vi "Final.vi"() -> ()   [LabVIEW 2013]
uses:
  <vilib>/DAQmx/read.llb/DAQmx Read (Analog Wfm 1Chan NSamp).vi
  <vilib>/DAQmx/miscellaneous.llb/DAQmx Fill In Error Info.vi
  <vilib>/express/express analysis/Spectral/Block/exnSpectralBlock spectral measurements PSD poly.vi
  <vilib>/express/express analysis/Spectral/Block/exnSpectralBlock spectral measurements PSD WFM.vi
  <vilib>/express/express analysis/Spectral/XNode/ExpressSpectralMeasurementsBlockNode.xnode
panel:
  in  "Signal de Reference":T1(ring)
  in  "Offset":dbl
  in  "Amplitude":dbl
  in  "Phase":dbl
  in  "Frequence 2":dbl
  in  "Voie physique DAQmx":tag="sHIT/ai0"
  in  "Statistiques":bool
  out "Moyenne":dbl
  out "Valeur eff":dbl
  out "Frequence":dbl
  in  "FFT":bool
  in  "Fenetre d'affichage (s)":dbl step=0.001
  out "Signal":waveform(dbl)[](graph)
  out "FFT":cluster{"f0":dbl, "df":dbl, "magnitude":dbl[]}(graph)
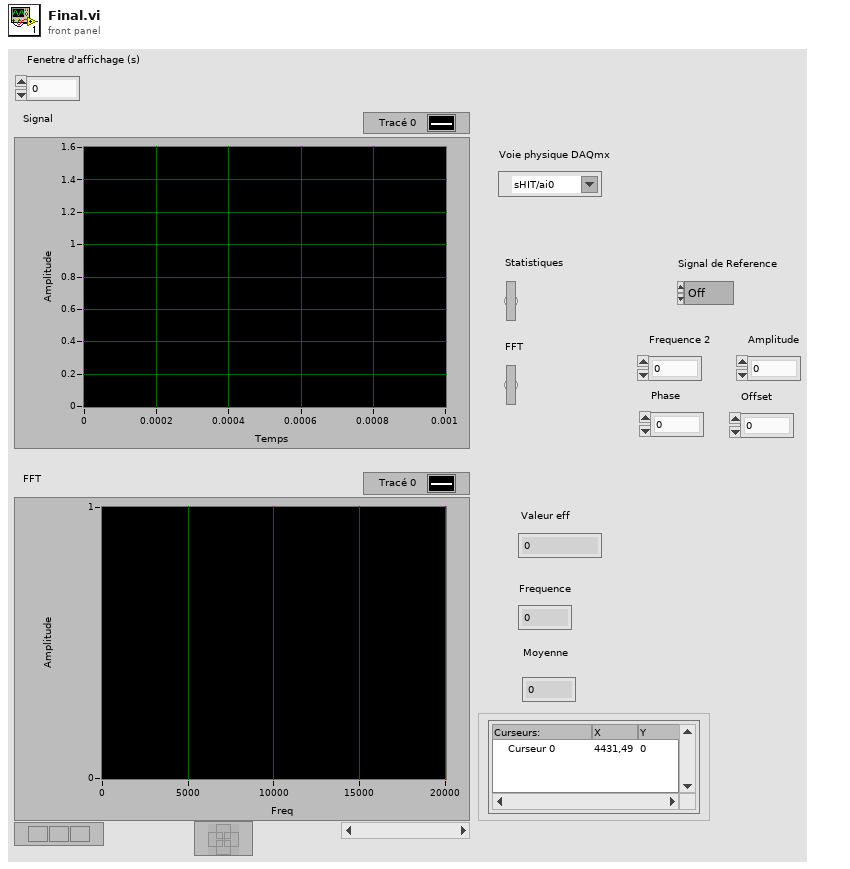
[diagram p1: front panel]
types:
  T1 = enum16{"Off", "Sinus", "Carre", "Triangle", "Scie"}
  T2 = enum16{"Off", "Sinus", "Carre", "Triangle", "Scie", ""}
  T3 = cluster{"averaging mode":u16, "weighting mode":u16, "number of averages":u32}
  T4 = cluster{"dB On (F)":bool, "unwrap phase (F)":bool, "convert to degree (F)":bool}
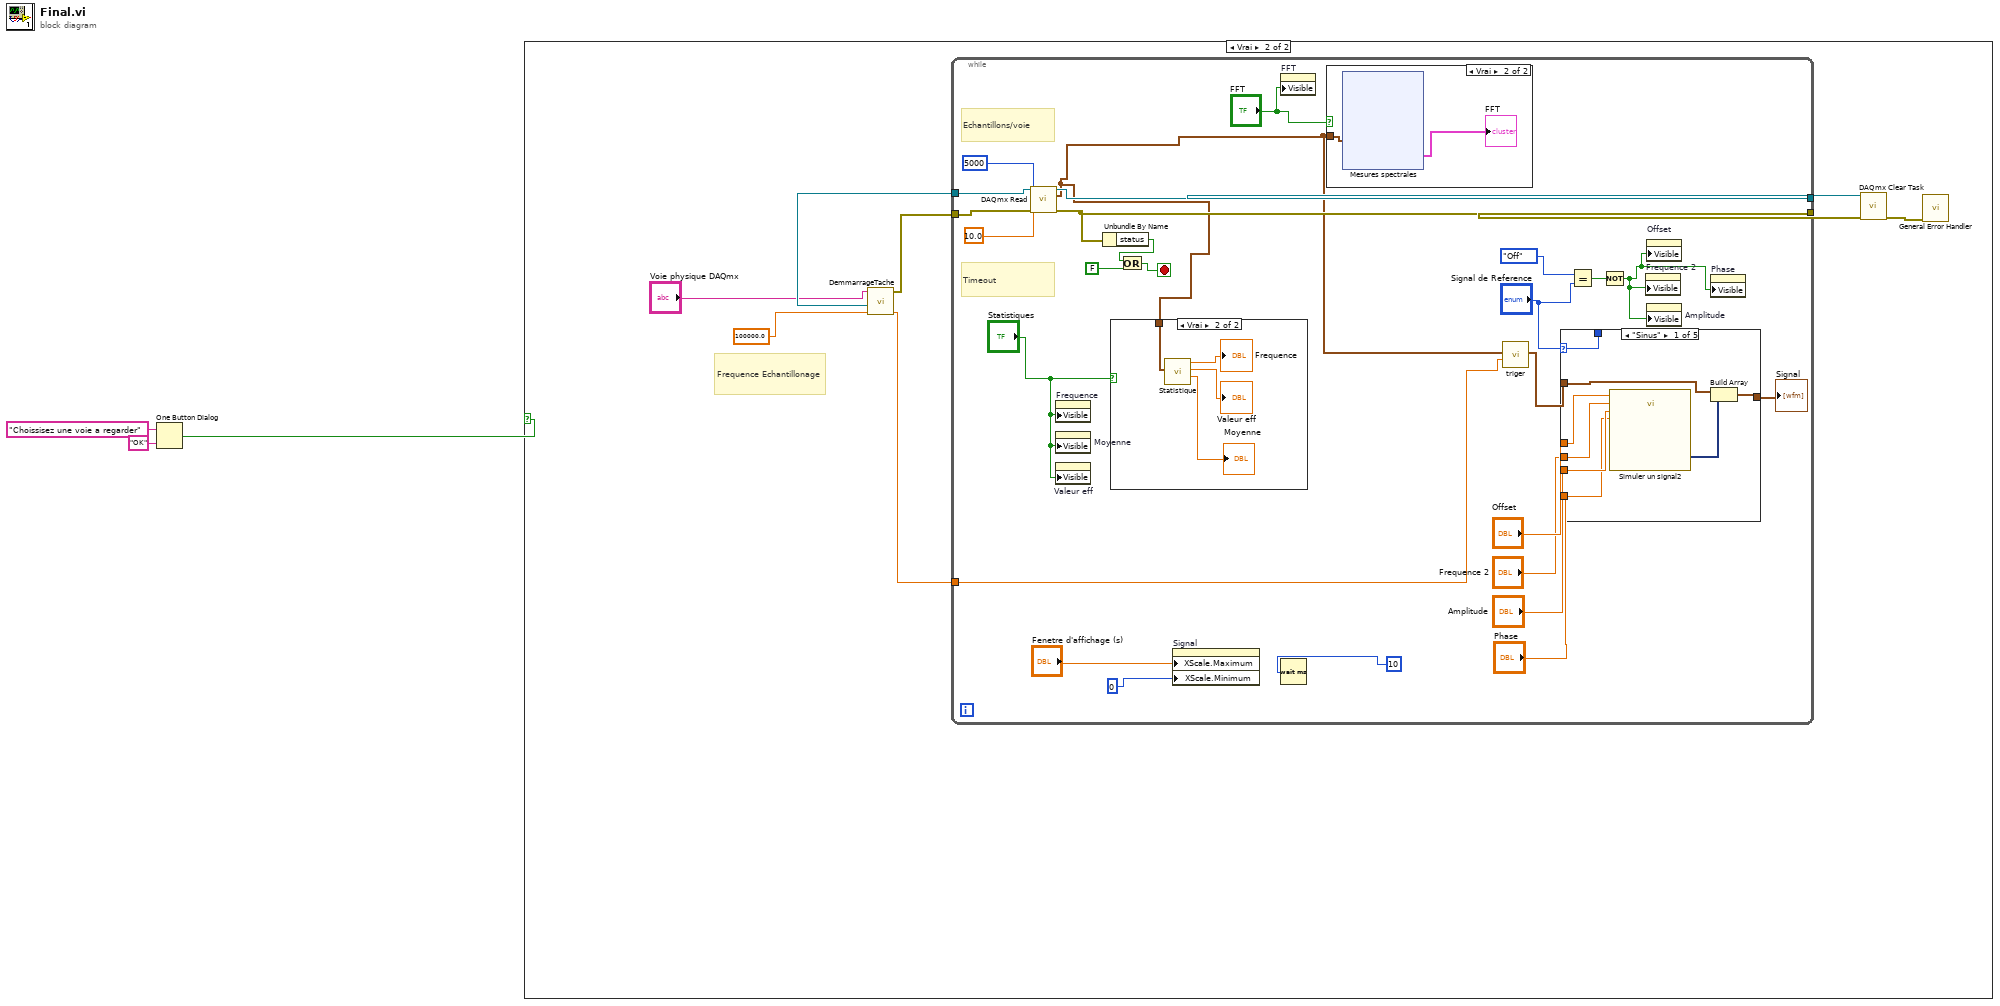
[diagram p0: block diagram]
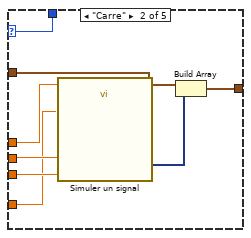
[diagram p3: hidden frame]
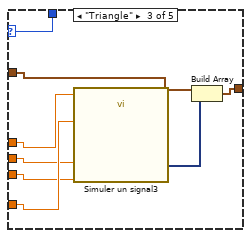
[diagram p4: hidden frame]
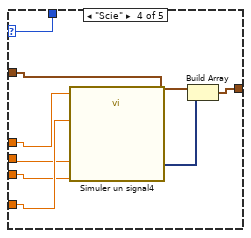
[diagram p5: hidden frame]
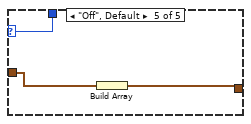
[diagram p6: hidden frame]
diagram:
  n1 = One Button Dialog(message="Choissisez une voie a regarder", button name ("OK")="OK" ("nom du bouton (\"OK\")")) -> (true=w1:bool)
  n2 = case shown="Vrai" w1 {
    frame False {
    }
    frame True {
      # "Frequence Echantillonage"
      n3 = call "DemmarrageTache.vi"("frequence echantillonage"=100000.0, "Voie physique DAQmx"="Voie physique DAQmx") -> ("frequence echantillonage 2"=w5:dbl, "task out"=w6:refnum<k21>, "error out"=w7:errorcluster)  [unwired: 6 in]
      n4 = while {
        tunnel: w6 -> [w37]
        tunnel: w7 -> [w36]
        tunnel: [w34] -> w11
        tunnel: [w30] -> w10
        tunnel: w5 -> [w22]
        stop <- w33 stop-if-true
        # "Echantillons/voie"
        # "Timeout"
        n5 = call-poly <vilib>:"DAQmx Read.vi"("task/channels in"=w37, "number of samples per channel"=5000, "timeout"=10.0, "error in"=w36) -> ("task out"=w34:refnum<k21>, "data"=w23:waveform(dbl), "error out"=w30:errorcluster)  [unwired: 9 in]
        n6 = property on="Frequence" class="NumNb (strict)"("Visible"="Statistiques") -> ()  [unwired: 2 in, 2 out]
        n7 = property on="Moyenne" class="NumNb (strict)"("Visible"="Statistiques") -> ()  [unwired: 2 in, 2 out]
        n8 = property on="Valeur eff" class="NumNb (strict)"("Visible"="Statistiques") -> ()  [unwired: 2 in, 2 out]
        n9 = Unbundle By Name(w30) -> ("status"=w31:bool)
        n10 = case shown="Vrai" "Statistiques" {
          tunnel: w23 -> [_ w76]
          frame False {
          }
          frame True {
            n11 = call "Statistique.vi"("Waveform"=w76) -> ("mean"=→"Moyenne":dbl, "Valeur efficace"=→"Valeur eff":dbl, "Fréquence"=→"Frequence":dbl)  [unwired: 8 in]
          }
        }
        n12 = Or(x=w31, y=FALSE) -> (x .or. y?=w33:bool)
        n13 = property on="Signal" class="GraphWF (strict)"("XScale.Maximum"="Fenetre d'affichage (s)", "XScale.Minimum"=0) -> ()  [unwired: 2 in, 2 out]
        n14 = property on="FFT" class="GraphWF (strict)"("Visible"="FFT") -> ()  [unwired: 2 in, 2 out]
        n15 = Wait (ms)(milliseconds to wait=10) -> ()  [unwired: 1 out]
        n16 = case shown="Vrai" "FFT" {
          tunnel: w23 -> [_ w77]
          frame False {
          }
          frame True {
            n17 = xnode "Mesures spectrales"("Signaux"=w77) -> ("DSP"=→"FFT":cluster{"f0":dbl, "df":dbl, "magnitude":dbl[]})  [unwired: 1 in, 1 out]
          }
        }
        n18 = call "triger.vi"("frequene echantillonage"=w22, "Signal"=w23) -> ("waveform en sortie"=w17:waveform(dbl))  [unwired: 9 in]
        n19 = case shown="\"Sinus\"" "Signal de Reference" {
          selector: "Signal de Reference" -> [w38 w46 w54 w62 w70]
          tunnel: "Offset" -> [w43 w53 w57 w65 _]
          tunnel: "Frequence 2" -> [w42 w52 w58 w66 _]
          tunnel: "Amplitude" -> [w41 w51 w59 w67 _]
          tunnel: "Phase" -> [w40 w50 w60 w68 _]
          tunnel: w17 -> [w39 w48 w56 w64 w72]
          tunnel: [w44 w47 w55 w63 w71] -> w16
          tunnel: [w38 w46 w54 w62 w70] -> _
          frame "Sinus" {
            n20 = call "Simuler un signal2"("Offset"=w43, "Frequency"=w42, "Amplitude"=w41, "Phase"=w40) -> ("Sinus"=w45:dynamicdata)  [unwired: 10 in, 1 out]
            n21 = Build Array(w39, w45) -> (w44:waveform(dbl)[])
          }
          frame "Carre" {
            n22 = call "Simuler un signal"("Offset"=w53, "Frequency"=w52, "Amplitude"=w51, "Phase"=w50) -> ("Carré"=w49:dynamicdata)  [unwired: 10 in, 1 out]
            n23 = Build Array(w48, w49) -> (w47:waveform(dbl)[])
          }
          frame "Triangle" {
            n24 = call "Simuler un signal3"("Offset"=w57, "Frequency"=w58, "Amplitude"=w59, "Phase"=w60) -> ("Triangle"=w61:dynamicdata)  [unwired: 10 in, 1 out]
            n25 = Build Array(w56, w61) -> (w55:waveform(dbl)[])
          }
          frame "Scie" {
            n26 = call "Simuler un signal4"("Offset"=w65, "Frequency"=w66, "Amplitude"=w67, "Phase"=w68) -> ("Dents de scie"=w69:dynamicdata)  [unwired: 10 in, 1 out]
            n27 = Build Array(w64, w69) -> (w63:waveform(dbl)[])
          }
          frame "Off", Default {
            n28 = Build Array(w72) -> (w71:waveform(dbl)[])
          }
        }
        "Signal" <- w16
        n29 = Equal?(x=T2."Off" ("Énum 2"), y="Signal de Reference") -> (x = y?=w13:bool)
        n30 = Not(x=w13) -> (.not. x?=w12:bool)
        n31 = property on="Frequence 2" class="NumNb (strict)"("Visible"=w12) -> ()  [unwired: 2 in, 2 out]
        n32 = property on="Offset" class="NumNb (strict)"("Visible"=w12) -> ()  [unwired: 2 in, 2 out]
        n33 = property on="Amplitude" class="NumNb (strict)"("Visible"=w12) -> ()  [unwired: 2 in, 2 out]
        n34 = property on="Phase" class="NumNb (strict)"("Visible"=w12) -> ()  [unwired: 2 in, 2 out]
      }
      n35 = call <vilib>:"DAQmx Clear Task.vi"("task in"=w11, "error in"=w10) -> ("error out"=w9:errorcluster)  [unwired: 13 in]
      n36 = call <vilib>:"General Error Handler.vi"("error in (no error)"=w9) -> ()  [unwired: 10 in, 5 out]
    }
  }
